vi "HexConvert.vi"(8 "E Field":string[](array[string]), 9 "Phase Field":string[](array[string]), 10 "Pockels_Galvo_Params":T1, 11 "Frequency Record":T2) -> (2 "Interrupted":bool, 3 "Hex":string)   [LabVIEW 2020]
uses:
  Controls/Frequency Record.ctl
  Controls/Pockels_Galvo_Params.ctl
  Global Variables/General Globals.vi
panel:
  out "Array":i32[](array[numeric])
  out "x-y":u32
  out "Numeric":i32
  # "RE-ENTRANT"
  # "SUBROUTINE"
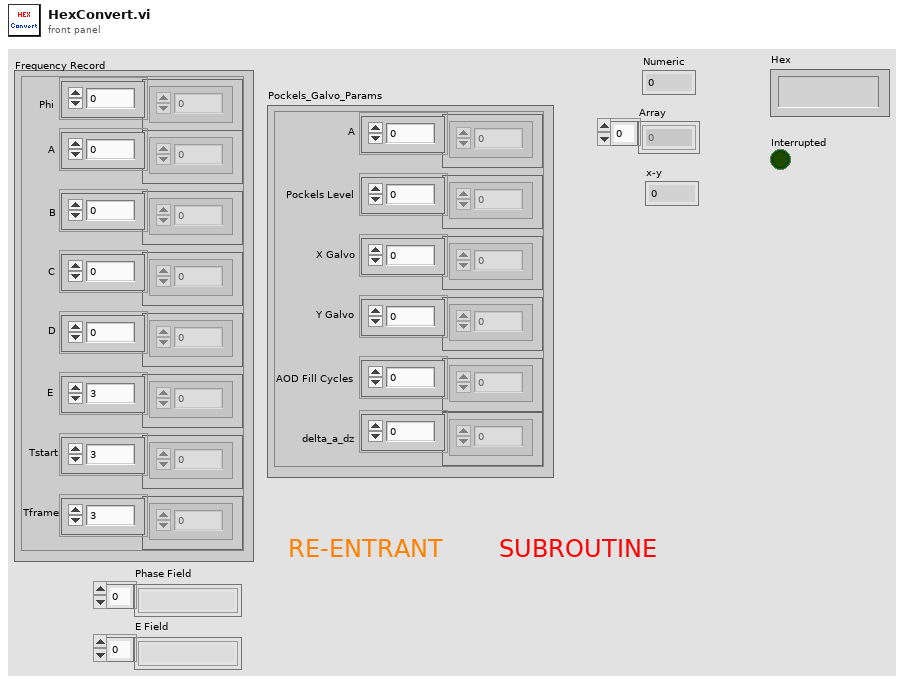
[diagram p1: front panel]
types:
  T1 = typedef "Pockels_Galvo_Params.ctl" = cluster{"A":dbl[], "Pockels Level":dbl[], "X Galvo":dbl[], "Y Galvo":dbl[], "AOD Fill Cycles":dbl[], "delta_a_dz":dbl[]}
  T2 = typedef "Frequency Record.ctl" = cluster{"Phi":dbl[], "A":dbl[], "B":dbl[], "C":dbl[], "D":dbl[], "E":dbl[], "Tstart":dbl[], "Tframe":dbl[]}
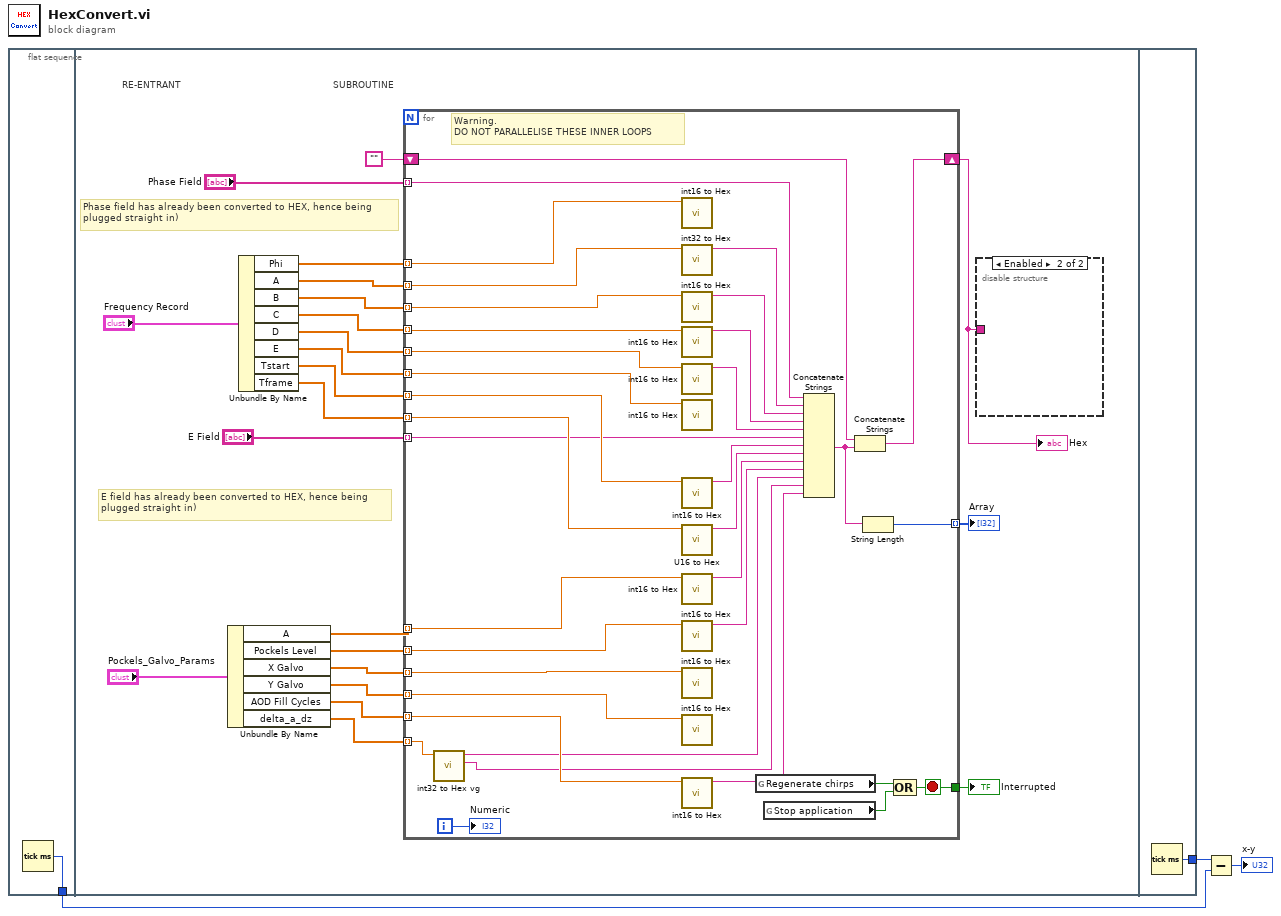
[diagram p0: block diagram]
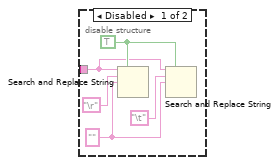
[diagram p2: hidden frame]
diagram:
  n1 = flat-sequence {
    tunnel: [w4] -> w2
    tunnel: [w67] -> w3
    frame #0 {
      n2 = Tick Count (ms)() -> (millisecond timer value=w4:u32)
    }
    frame #1 {
      # "Phase field has already been converted to HEX, hence being\nplugged straight in)"
      # "E field has already been converted to HEX, hence being\nplugged straight in)"
      # "SUBROUTINE"
      # "RE-ENTRANT"
      n3 = Unbundle By Name("Pockels_Galvo_Params") -> ("A"=w25:dbl[], "Pockels Level"=w24:dbl[], "X Galvo"=w23:dbl[], "Y Galvo"=w22:dbl[], "AOD Fill Cycles"=w15:dbl[], "delta_a_dz"=w6:dbl[])
      n4 = Unbundle By Name("Frequency Record") -> ("Phi"=w26:dbl[], "A"=w14:dbl[], "B"=w21:dbl[], "C"=w20:dbl[], "D"=w19:dbl[], "E"=w18:dbl[], "Tstart"=w17:dbl[], "Tframe"=w16:dbl[])
      n5 = for {
        tunnel: w26 -> [w65] mode=indexing
        tunnel: w25 -> [w56] mode=indexing
        tunnel: w24 -> [w54] mode=indexing
        tunnel: w23 -> [w53] mode=indexing
        tunnel: w22 -> [w48] mode=indexing
        tunnel: w14 -> [w64] mode=indexing
        tunnel: w21 -> [w62] mode=indexing
        tunnel: w20 -> [w61] mode=indexing
        tunnel: w19 -> [w60] mode=indexing
        tunnel: w18 -> [w58] mode=indexing
        tunnel: w17 -> [w46] mode=indexing
        tunnel: w16 -> [w44] mode=indexing
        tunnel: w15 -> [w51] mode=indexing
        shift-right: [w47] -> w10
        shift-left: "" -> [w42]
        tunnel: [w39] -> w9
        tunnel: "Phase Field" -> [w38] mode=indexing
        tunnel: "E Field" -> [w37] mode=indexing
        tunnel: w6 -> [w36] mode=indexing
        tunnel: [w32] -> w5 mode=indexing
        i -> [w45]
        stop <- w39 stop-if-true
        # "Warning.\nDO NOT PARALLELISE THESE INNER LOOPS"
        n6 = call "int32 to Hex vg.vi"("number"=w36) -> ("[31:16]"=w34:string, "[15:0]"=w35:string)  [unwired: 8 in, 1 out]
        n7 = call "int16 to Hex.vi"("number"=w65) -> ()  [unwired: 10 in, 1 out]
        n8 = call "int32 to Hex.vi"("number"=w64) -> ("Hex string"=w66:string)  [unwired: 10 in]
        n9 = call "int16 to Hex.vi"("number"=w62) -> ("Hex string"=w63:string)  [unwired: 10 in]
        n10 = call "int16 to Hex.vi"("number"=w61) -> ("Hex string"=w50:string)  [unwired: 10 in]
        n11 = call "int16 to Hex.vi"("number"=w60) -> ("Hex string"=w59:string)  [unwired: 10 in]
        n12 = call "int16 to Hex.vi"("number"=w58) -> ()  [unwired: 10 in, 1 out]
        n13 = call "int16 to Hex.vi"("number"=w46) -> ("Hex string"=w49:string)  [unwired: 10 in]
        n14 = call "U16 to Hex.vi"("number"=w44) -> ("Hex string"=w43:string)  [unwired: 10 in]
        n15 = call "int16 to Hex.vi"("number"=w56) -> ("Hex string"=w57:string)  [unwired: 10 in]
        n16 = call "int16 to Hex.vi"("number"=w54) -> ("Hex string"=w55:string)  [unwired: 10 in]
        n17 = call "int16 to Hex.vi"("number"=w53) -> ()  [unwired: 10 in, 1 out]
        n18 = call "int16 to Hex.vi"("number"=w48) -> ()  [unwired: 10 in, 1 out]
        n19 = call "int16 to Hex.vi"("number"=w51) -> ("Hex string"=w52:string)  [unwired: 10 in]
        n20 = global read "General Globals.vi" "Regenerate chirps"() -> (w40:bool)
        n21 = global read "General Globals.vi" "Stop application"() -> (w41:bool)
        n22 = Concatenate Strings(w38, w66, w63, w50, w59, w37, w49, w43, w57, w55, w35, w34, w52) -> (w33:string)
        n23 = Concatenate Strings(w42, w33) -> (w47:string)
        n24 = String Length(string=w33) -> (length=w32:i32)
        n25 = Compound Arithmetic op=OR(w40, w41) -> (w39:bool)
        "Numeric" <- w45
      }
      "Hex" <- w10
      "Interrupted" <- w9
      "Array" <- w5
      n26 = disable-structure shown="Enabled" {
        disable-tunnel: w10 -> [w27 _]
        frame Disabled {
          w29 = TRUE
          w28 = "" ("replace string (\"\")")
          n27 = Search and Replace String(replace all?=w29, input string=w27, search string="\r", replace string=w28) -> ()  [unwired: 4 in, 4 out]
          n28 = Search and Replace String(replace all?=w29, input string=w27, search string="\t", replace string=w28) -> ()  [unwired: 4 in, 4 out]
        }
        frame Enabled {
        }
      }
    }
    frame #2 {
      n29 = Tick Count (ms)() -> (millisecond timer value=w67:u32)
    }
  }
  n30 = Subtract(x=w3, y=w2) -> (x-y=→"x-y":u32)
